vi "Read SequenceIndices.vi"(8 "error in (no error)":errorcluster, 11 "VariableManager in":refnum<class "VariableManager.lvclass">) -> (0 "error out":errorcluster, 2 "SequenceIndices":refnum<class "SequenceIndex.lvclass">[](array[class]), 3 "VariableManager out":refnum<class "VariableManager.lvclass">)   [LabVIEW 2013, in "VariableManager.lvclass"]
uses:
  VariableManager.lvclass
  SequenceIndex/SequenceIndex.lvclass
  VariableManager.lvclass/VariableManager.ctl
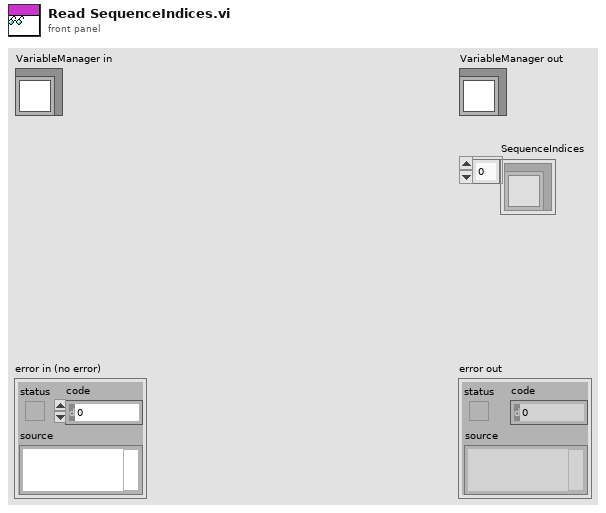
[diagram p1: front panel]
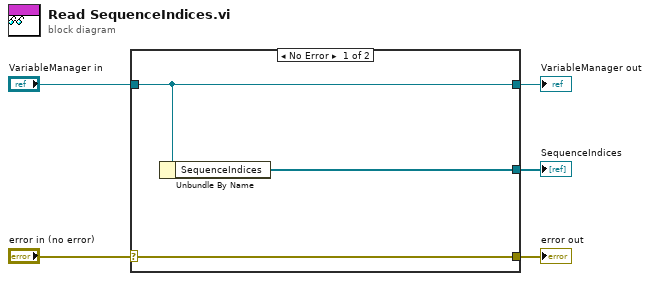
[diagram p0: block diagram]
diagram:
  n1 = case shown="No Error" "error in (no error)" {
    selector: "error in (no error)" -> [w8 w9]
    tunnel: [w8 w9] -> w4
    tunnel: [w7 w10] -> w2
    tunnel: "VariableManager in" -> [w7 w10]
    tunnel: [w6 _] -> w1
    frame No Error {
      n2 = Unbundle By Name(w7) -> ("SequenceIndices"=w6:refnum<class "SequenceIndex.lvclass">[])
    }
    frame Error {
    }
  }
  "error out" <- w4
  "VariableManager out" <- w2
  "SequenceIndices" <- w1
